vi "Move VIs.vi"(8 "error in (no error)":errorcluster, 10 "VIs to Move":path[](array[path]), 11 "Destination":path) -> (0 "error out":errorcluster)   [LabVIEW 2020, in "Mock Class Updater.lvclass"]
uses:
  Mock Class Updater.lvclass
  Mock Class Updater.lvclass/Mock Class Updater.ctl
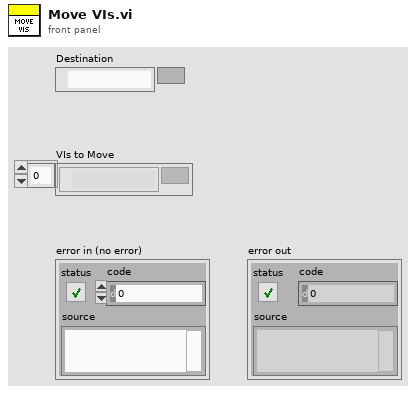
[diagram p1: front panel]
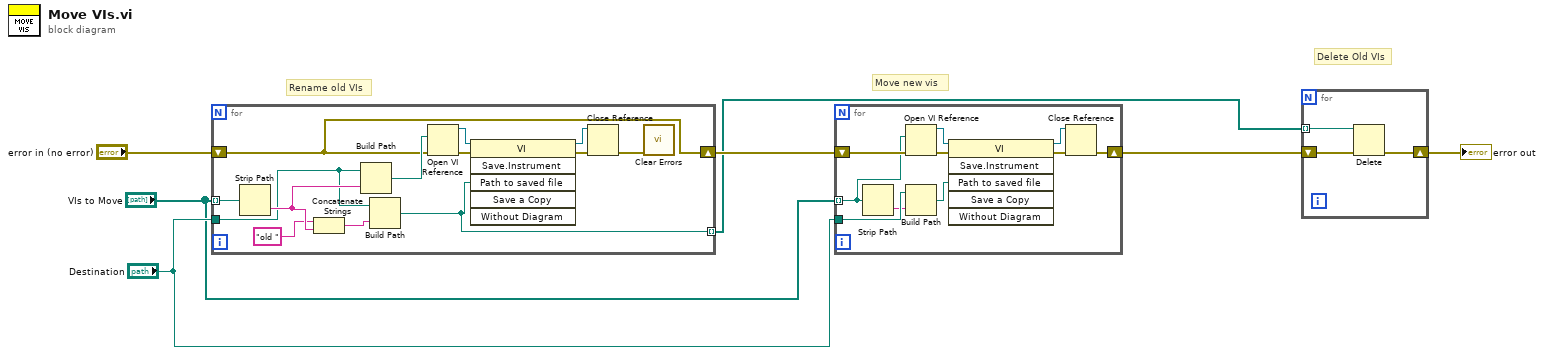
[diagram p0: block diagram]
diagram:
  # "Delete Old VIs"
  # "Move new vis"
  # "Rename old VIs"
  n1 = for {
    shift-right: [w8] -> w6
    shift-left: "error in (no error)" -> [w8]
    tunnel: "VIs to Move" -> [w18] mode=indexing
    tunnel: "Destination" -> [w11]
    tunnel: [w9] -> w5 mode=indexing
    n2 = Strip Path(path=w18) -> (name=w13:string)  [unwired: 1 out]
    n3 = Concatenate Strings("old " ("string"), w13) -> (w10:string)
    n4 = Build Path(base path=w11, name or relative path=w13) -> (appended path=w14:path)
    n5 = Build Path(base path=w11, name or relative path=w10) -> (appended path=w9:path)
    n6 = Open VI Reference(vi path=w14, error in (no error)=w8) -> (vi reference=w17:refnum<vi>, error out=w19:errorcluster)  [unwired: 4 in]
    n7 = invoke class="VI" method="Save.Instrument"(reference=w17, error in=w19, "Path to saved file"=w9) -> (reference out=w15:refnum<vi>, error out=w20:errorcluster)  [unwired: 3 in, 4 out]
    n8 = Close Reference(reference=w15, error in (no error)=w20) -> (error out=w16:errorcluster)
    n9 = call <vilib>:"Clear Errors.vi"("error in (no error)"=w16) -> ()  [unwired: 5 in, 2 out]
  }
  n10 = for {
    shift-right: [w22] -> w7
    shift-left: w6 -> [w30]
    tunnel: "VIs to Move" -> [w27] mode=indexing
    tunnel: "Destination" -> [w25]
    n11 = Strip Path(path=w27) -> (name=w24:string)  [unwired: 1 out]
    n12 = Open VI Reference(vi path=w27, error in (no error)=w30) -> (vi reference=w26:refnum<vi>, error out=w28:errorcluster)  [unwired: 4 in]
    n13 = Build Path(base path=w25, name or relative path=w24) -> (appended path=w23:path)
    n14 = invoke class="VI" method="Save.Instrument"(reference=w26, error in=w28, "Path to saved file"=w23) -> (reference out=w21:refnum<vi>, error out=w29:errorcluster)  [unwired: 3 in, 4 out]
    n15 = Close Reference(reference=w21, error in (no error)=w29) -> (error out=w22:errorcluster)
  }
  n16 = for {
    shift-right: [w32] -> w3
    shift-left: w7 -> [w33]
    tunnel: w5 -> [w31] mode=indexing
    n17 = Delete(path (use dialog)=w31, error in=w33) -> (error out=w32:errorcluster)  [unwired: 3 in, 2 out]
  }
  "error out" <- w3
